vi "Try Match Response.vi"(8 "error in":errorcluster, 10 "ICAN CC Frame":refnum<class "ICAN CC Frame.lvclass">, 11 "Block Upload Transfer in":refnum<class "Block Upload Sub-Block Transfer.lvclass">) -> (0 "error out":errorcluster, 2 "Match":bool, 3 "SDO Transfer out":refnum<class "SDO Transfer.lvclass">)   [LabVIEW 2020, in "CANopen.lvlib" / "SDO Manager.lvlib" / "Block Upload Sub-Block Transfer.lvclass"]
uses:
  Block Upload Sub-Block Transfer.lvclass
  D:/git/CANopen-LabVIEW/source/SDO/SDO Manager/SDO Transfer/SDO Transfer.lvclass
  SDO Transfer/SDO Transfer.lvclass
  HAL/Source/Interfaces/ICAN CC Frame/ICAN CC Frame.lvclass
  D:/git/HAL/Source/Interfaces/IMessage/IMessage.lvclass
  SDO Transfer/SDO Transfer.lvclass/SDO Transfer.ctl
  Block Upload Sub-Block Transfer.lvclass/Block Upload Sub-Block Transfer.ctl
  Block Upload End Transfer/Block Upload End Transfer.lvclass
  HAL/Source/Interfaces/ICommunicate/ICommunicate.lvclass
  CANopen Message/CANopen Message.lvclass
  SDO Transfer/SDO abort code.ctl
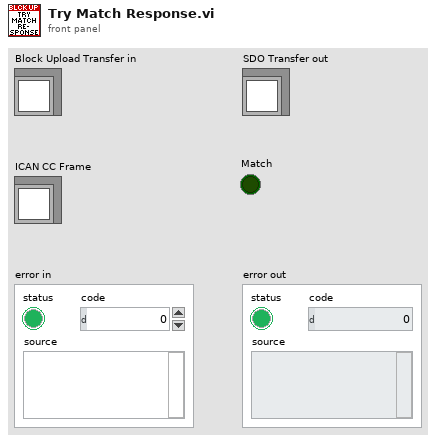
[diagram p1: front panel]
types:
  T1 = typedef "CANopen.lvlib/SDO Manager.lvlib/SDO Transfer.lvclass/SDO abort code.ctl" = u32
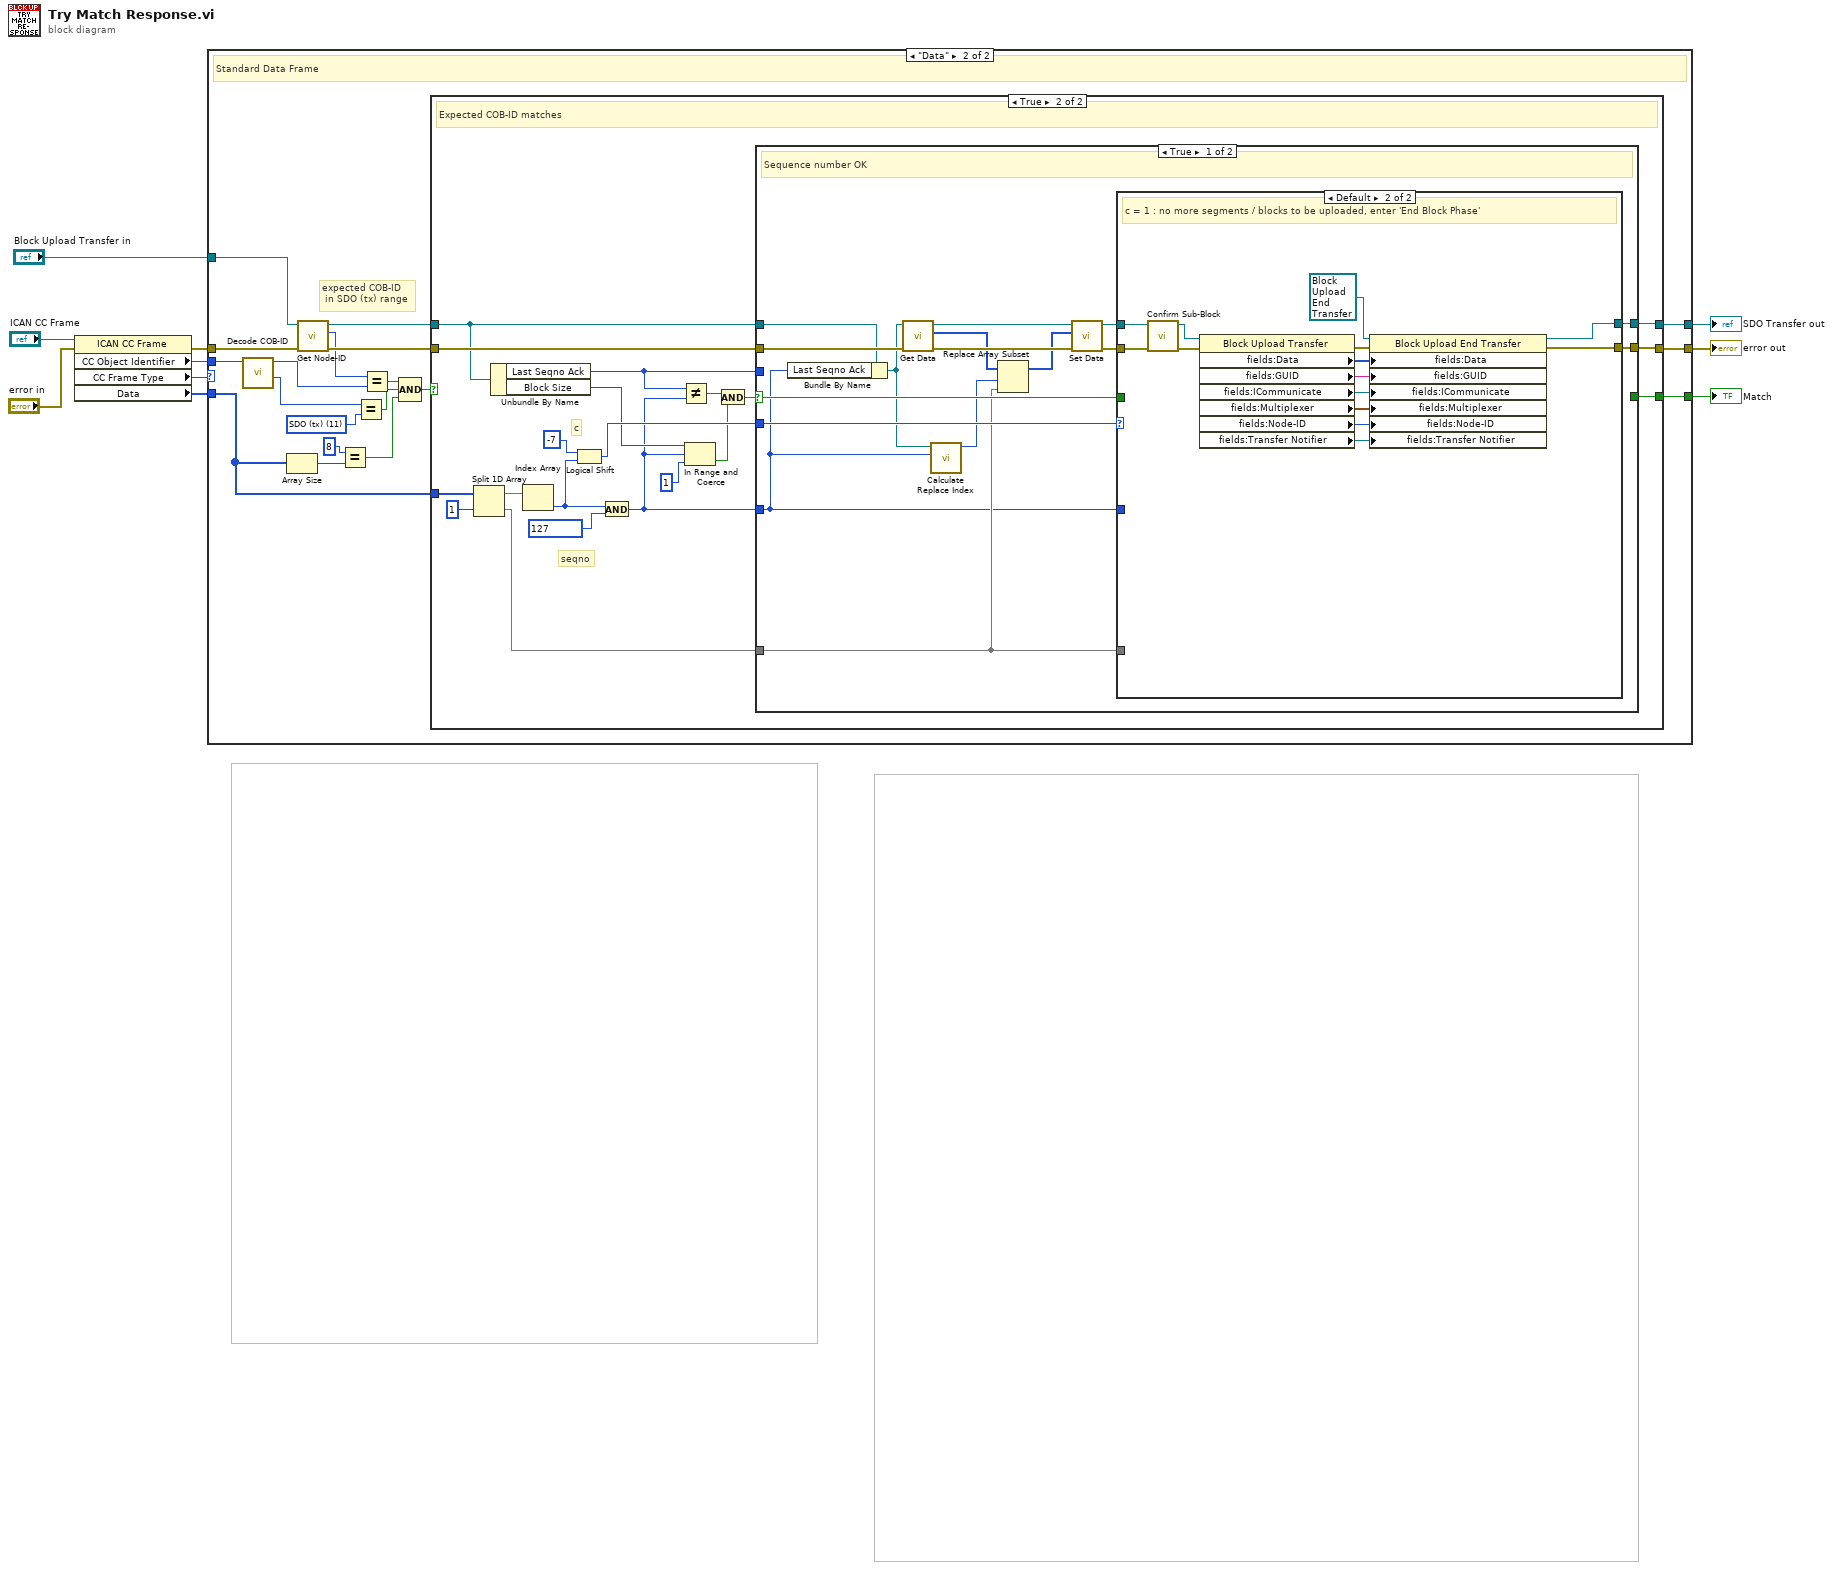
[diagram p0: block diagram]
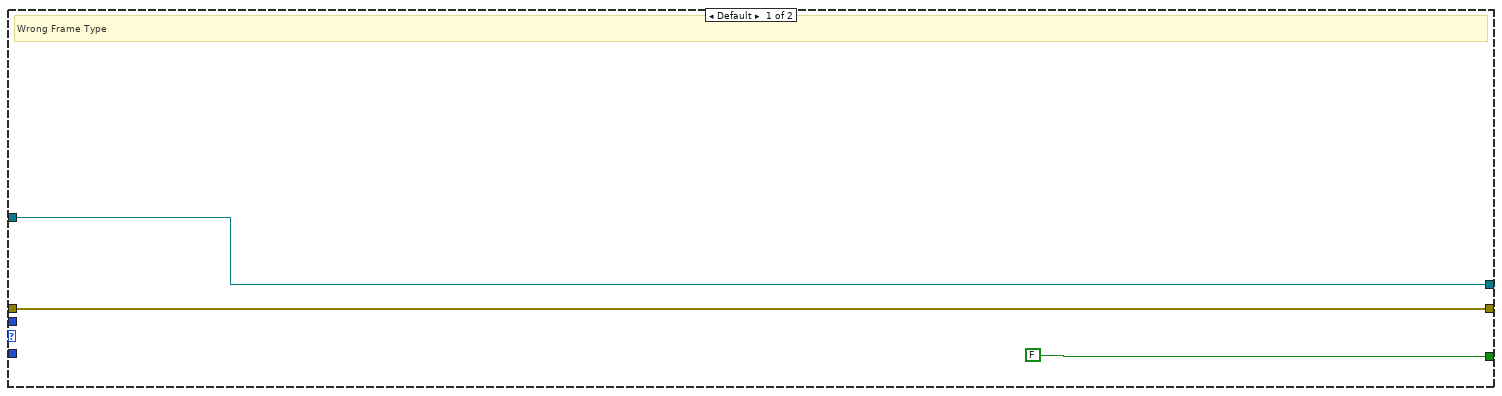
[diagram p2: hidden frame]
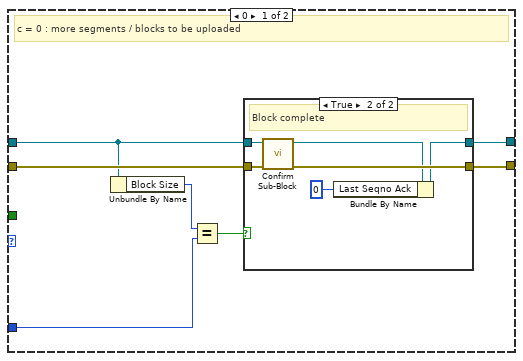
[diagram p4: hidden frame]
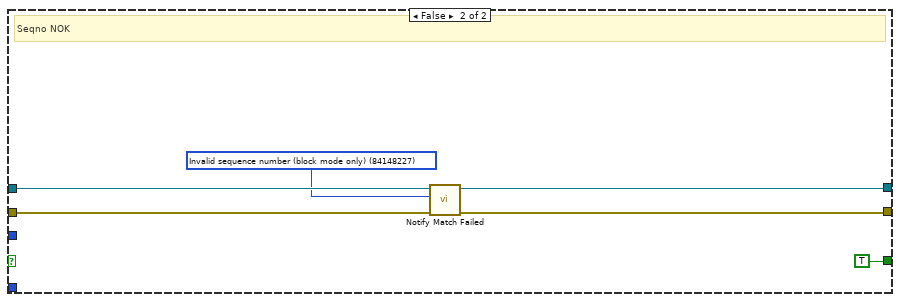
[diagram p6: hidden frame]
diagram:
  n1 = property class="ICAN CC Frame"(reference="ICAN CC Frame", error in="error in") -> (error out=w9:errorcluster, "CC Object Identifier"=w8:u32, "CC Frame Type"=w6:enum8{"Data", "Remote", "Error", "Overload"}, "Data"=w7:u8[])  [unwired: 1 out]
  n2 = case shown="\"Data\"" w6 {
    tunnel: w9 -> [w12 w32]
    tunnel: "Block Upload Transfer in" -> [w11 w31]
    tunnel: [w11 w28] -> w2
    tunnel: [w12 w27] -> w10
    tunnel: [FALSE w26] -> w1
    tunnel: w8 -> [_ w25]
    tunnel: w7 -> [_ w14]
    frame Default {
      # "Wrong Frame Type"
    }
    frame "Data" {
      w22 = u8 11 items=["NMT"=0, "EMCY/SYNC"=1, "TIME"=2, "PDO1 (tx)"=3, "PDO1 (rx)"=4, "PDO2 (tx)"=5, "PDO2 (rx)"=6, "PDO3 (tx)"=7, "PDO3 (rx)"=8, "PDO4 (tx)"=9, "PDO4 (rx)"=10, "SDO (tx)"=11, "SDO (rx)"=12, "NMT error control"=14] ("Function Code")
      # "expected COB-ID\n in SDO (tx) range"
      # "Standard Data Frame"
      n3 = call "Decode COB-ID.vi"("COD-ID"=w25) -> ("Function Code"=w21:u8, "Node-ID"=w24:u8)  [unwired: 9 in]
      n4 = Array Size(array=w14) -> (size(s)=w20:i32)
      n5 = call "Get Node-ID.vi"("error in"=w32, "SDO Transfer in"=w31) -> ("error out"=w29:errorcluster, "Node-ID"=w23:u8, "SDO Transfer out"=w30:refnum<class "Block Upload Sub-Block Transfer.lvclass">)  [unwired: 7 in]
      n6 = Equal?(x=8, y=w20) -> (x = y?=w15:bool)
      n7 = Equal?(x=w21, y=w22) -> (x = y?=w16:bool)
      n8 = Equal?(x=w23, y=w24) -> (x = y?=w17:bool)
      n9 = Compound Arithmetic op=AND(w17, w16, w15) -> (w18:bool)
      n10 = case shown="True" w18 {
        tunnel: w30 -> [w34 w42]
        tunnel: w29 -> [w33 w53]
        tunnel: [w34 w49] -> w28
        tunnel: [w33 w50] -> w27
        tunnel: w14 -> [_ w51]
        tunnel: [_ w48] -> w26
        frame False {
          # "COB-ID mismatch"
        }
        frame True {
          # "seqno"
          # "c"
          # "Expected COB-ID matches"
          n11 = Split 1D Array(array=w51, index=1) -> (first subarray=w45:u8[], second subarray=w46:u8[])
          n12 = Unbundle By Name(w42) -> ("Last Seqno Ack"=w40:u8, "Block Size"=w38:u8)
          n13 = Index Array(array=w45) -> (element=w43:u8)  [unwired: 1 in]
          n14 = Logical Shift(y=i16 -7, x=w43) -> (x << y=w52:u8)
          n15 = And(x=w43, y=u8 127 ("seqno")) -> (x .and. y?=w37:u8)
          n16 = Not Equal?(x=w40, y=w37) -> (x != y?=w41:bool)
          n17 = In Range and Coerce(upper limit=w38, x=w37, lower limit=u8 1) -> (In Range?=w35:bool)  [unwired: 1 out]
          n18 = And(x=w41, y=w35) -> (x .and. y?=w36:bool)
          n19 = case shown="True" w36 {
            selector: w36 -> [w66 _]
            tunnel: w53 -> [w70 w105]
            tunnel: w52 -> [w69 _]
            tunnel: [w68 w104] -> w50
            tunnel: [w67 w102] -> w49
            tunnel: [_ TRUE] -> w48
            tunnel: w46 -> [w57 _]
            tunnel: w42 -> [w59 w103]
            tunnel: w37 -> [w56 _]
            tunnel: w40 -> [_ _]
            frame True {
              # "Sequence number OK"
              n20 = Bundle By Name(cluster=w59, "Last Seqno Ack"=w56) -> (w58:refnum<class "Block Upload Sub-Block Transfer.lvclass">)
              n21 = call "Get Data.vi"("error in"=w70, "SDO Transfer in"=w58) -> ("error out"=w65:errorcluster, "Data"=w61:u8[], "SDO Transfer out"=w63:refnum<class "Block Upload Sub-Block Transfer.lvclass">)  [unwired: 7 in]
              n22 = call "Calculate Replace Index.vi"("Seqno"=w56, "Block Upload Transfer in"=w58) -> ("Replace Index"=w60:u8)  [unwired: 9 in]
              n23 = Replace Array Subset(array=w61, new element=w57, index=w60) -> (w55:u8[])
              n24 = call "Set Data.vi"("error in"=w65, "Data"=w55, "SDO Transfer in"=w63) -> ("error out"=w64:errorcluster, "SDO Transfer out"=w62:refnum<class "Block Upload Sub-Block Transfer.lvclass">)  [unwired: 7 in]
              n25 = case shown="Default" w69 {
                tunnel: w62 -> [w74 w88]
                tunnel: w64 -> [w77 w99]
                tunnel: [w75 w90] -> w67
                tunnel: [w76 w97] -> w68
                tunnel: w57 -> [_ _]
                tunnel: w66 -> [_ _]
                tunnel: w56 -> [w72 _]
                frame 0 {
                  # "c = 0 : more segments / blocks to be uploaded"
                  n26 = Unbundle By Name(w74) -> ("Block Size"=w73:u8)
                  n27 = Equal?(x=w73, y=w72) -> (x = y?=w71:bool)
                  n28 = case shown="True" w71 {
                    tunnel: w77 -> [w78 w85]
                    tunnel: [w78 w84] -> w76
                    tunnel: [w79 w81] -> w75
                    tunnel: w74 -> [w79 w82]
                    frame False {
                      # "Block incomplete"
                    }
                    frame True {
                      # "Block complete"
                      n29 = call "Confirm Sub-Block.vi"("error in"=w85, "Block Upload Transfer in"=w82) -> ("error out"=w84:errorcluster, "Block Upload Transfer out"=w83:refnum<class "Block Upload Sub-Block Transfer.lvclass">)  [unwired: 8 in]
                      n30 = Bundle By Name(cluster=w83, "Last Seqno Ack"=u8 0) -> (w81:refnum<class "Block Upload Sub-Block Transfer.lvclass">)
                    }
                  }
                }
                frame Default {
                  # "c = 1 : no more segments / blocks to be uploaded, enter 'End Block Phase'"
                  n31 = call "Confirm Sub-Block.vi"("error in"=w99, "Block Upload Transfer in"=w88) -> ("error out"=w89:errorcluster, "Block Upload Transfer out"=w87:refnum<class "Block Upload Sub-Block Transfer.lvclass">)  [unwired: 8 in]
                  n32 = property class="Block Upload Transfer"(reference=w87, error in=w89) -> (error out=w96:errorcluster, "fields:Data"=w86:u8[], "fields:GUID"=w95:string, "fields:ICommunicate"=w94:refnum<class "ICommunicate.lvclass">, "fields:Multiplexer"=w93:cluster{"Index":u16, "Sub-Index":u8}, "fields:Node-ID"=w92:u8, "fields:Transfer Notifier"=w91:refnum<notifier>)  [unwired: 1 out]
                  n33 = property class="Block Upload End Transfer"(reference=refnum<class "Block Upload End Transfer.lvclass"> refnum ("CANopen.lvlib:SDO Manager.lvlib:Block Upload End Transfer"), error in=w96, "fields:Data"=w86, "fields:GUID"=w95, "fields:ICommunicate"=w94, "fields:Multiplexer"=w93, "fields:Node-ID"=w92, "fields:Transfer Notifier"=w91) -> (reference out=w90:refnum<class "Block Upload End Transfer.lvclass">, error out=w97:errorcluster)
                }
              }
            }
            frame False {
              w101 = T1 84148227 items=["Toggle bit not allowed"=84082688, "SDO protocol timed out"=84148224, "Client/server command specifier not valid or unknown"=84148225, "Invalid block size (block mode only)"=84148226, "Invalid sequence number (block mode only)"=84148227, "CRC error (block mode only)"=84148228, "Out of memory"=84148229, "Attempt to read a write only object"=100728833, "Attempt to write a read only object"=100728834, "Object does not exist in the object dictionary"=100794368, "Object cannot be mapped to the PDO"=100925505, "The number and length of the objects to be mapped would exceed PDO length"=100925506, "General parameter incompatibility reason"=100925507, "General internal incompatibility in the device"=100925511, "Access failed due to an hardware error"=101056512, "Data type does not match, length of service parameter does not match"=101122064, "Data type does not match, length of service parameter too high"=101122066, "Data type does not match, length of service parameter too low"=101122067, "Sub-index does not exist"=101253137, "Invalid value for parameter (download only)"=101253168, "Value of parameter written too high (download only)"=101253169, "Value of parameter written too low (download only)"=101253170, "Maximum value is less than minimum value"=101253174, "Resource not available: SDO connection"=101318691, "General error"=134217728, "Data cannot be transferred or stored to the application"=134217760, "Data cannot be transferred or stored to the application because of local control"=134217761, "Data cannot be transferred or stored to the application because of the present device stable"=134217762, "Object dictionary dynamic generation fails or no object dictionary is present (e.g. object dictionary is generated from file and generation fails because of an file error)"=134217763, "No data available"=134217764] ("SDO abort code")
              # "Seqno NOK"
              n34 = call "Notify Match Failed.vi"("error in"=w105, "SDO abort code"=w101, "SDO Transfer in"=w103) -> ("error out"=w104:errorcluster, "SDO Transfer out"=w102:refnum<class "Block Upload Sub-Block Transfer.lvclass">)  [unwired: 7 in]
            }
          }
        }
      }
    }
  }
  "SDO Transfer out" <- w2
  "error out" <- w10
  "Match" <- w1
